vi "Write SSH Command.vi"(6 "Response Configuration":T2, 7 "Connection Name":string, 8 "error in (no error)":errorcluster, 9 "Command":string, 10 "Module ID":i32=-1, 11 "wait for reply (T)":bool=TRUE) -> (0 "error out":errorcluster, 1 "timed out?":bool, 2 "Reply Payload":T1)   [LabVIEW 2017]
doc: "Writes a command out to the module specified by Module ID or Connection Name.\nUse Response Configuration to determine how the module should send back a response."
uses:
  Response Configuration.ctl
  Libraries/SSH/SSH.lvlib
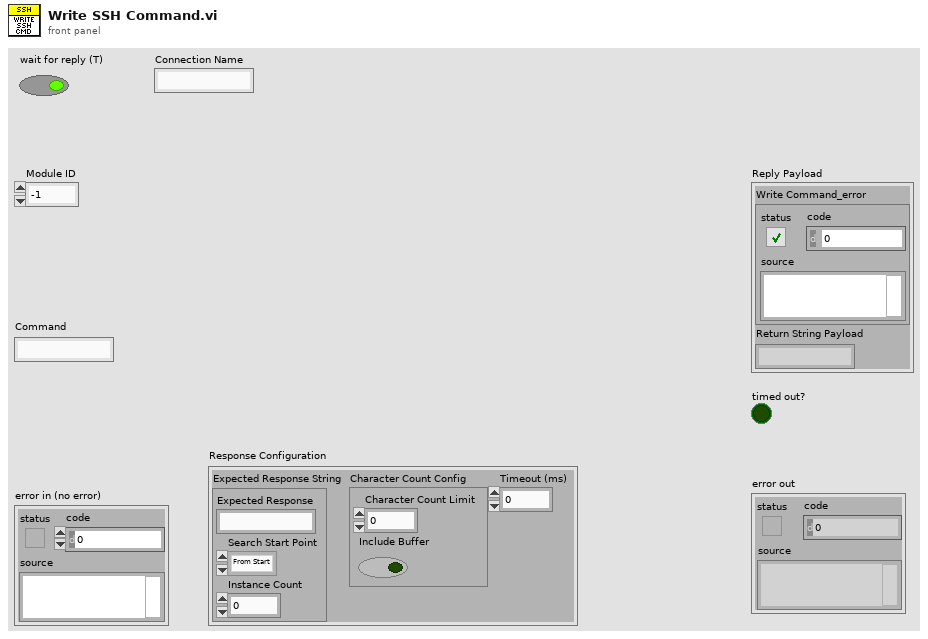
[diagram p1: front panel]
types:
  T1 = cluster{"Write Command_error":errorcluster, "Return String Payload":string}
  T2 = typedef "Response Configuration.ctl" = cluster{"Expected Response String":cluster{"Expected Response":string, "Search Start Point":enum16{"From Start", "From End"}, "Instance Count":i32}, "Character Count Config":cluster{"Character Count Limit":i32, "Include Buffer":bool}, "Timeout (ms)":i32}
  T3 = typedef "SSH.lvlib/Write Command (Reply Payload)--cluster.ctl" = cluster{"Write Command_error":errorcluster, "Return String Payload":string}
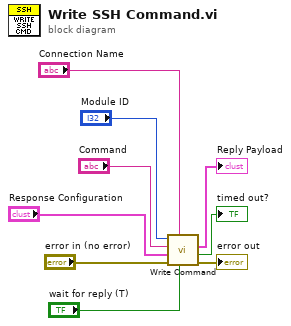
[diagram p0: block diagram]
diagram:
  n1 = call "Write Command.vi"("wait for reply (T)"="wait for reply (T)", "Connection Name"="Connection Name", "error in (no error)"="error in (no error)", "Response Configuration"="Response Configuration", "Command"="Command", "Module ID"="Module ID") -> ("error out"=→"error out":errorcluster, "timed out?"=→"timed out?":bool, "Reply Payload"=→"Reply Payload":T3)  [unwired: 3 in]
